vi "Write name.vi"(8 "error in":errorcluster, 10 "name":string, 11 "PL_Local Target Configuration in":refnum<class "PL_Target Configuration.lvclass">) -> (0 "error out":errorcluster, 3 "PL_Local Target Configuration out":refnum<class "PL_Target Configuration.lvclass">)   [LabVIEW 2013, in "PL_Target Configuration.lvclass"]
uses:
  PL_Target Configuration.lvclass
  PL_Target Configuration.lvclass/PL_Target Configuration.ctl
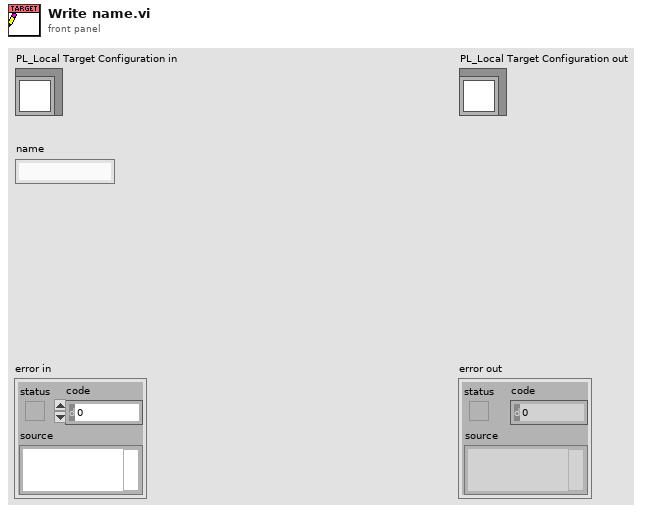
[diagram p1: front panel]
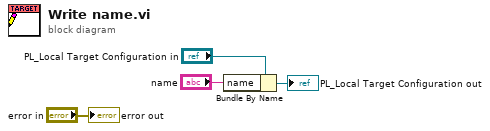
[diagram p0: block diagram]
diagram:
  n1 = Bundle By Name(cluster="PL_Local Target Configuration in", "name"="name") -> (→"PL_Local Target Configuration out":refnum<class "PL_Target Configuration.lvclass">)
  "error out" <- "error in"
